vi "X_Limit_Length_Key_Down.vi"(1 "Max String Length":i32, 2 "Char":i16, 3 "Input String":string) -> (0 "Discard?":bool)   [LabVIEW 2012, in "String_XControl.xctl"]
doc: "This code takes in the last char pressed, the maximum string length, and the current string. The output is a boolean that indicates whether or not to discard the last key press."
uses:
  String_XControl.xctl
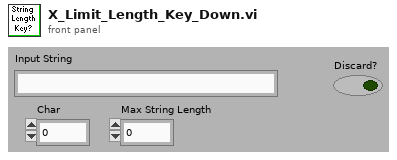
[diagram p1: front panel]
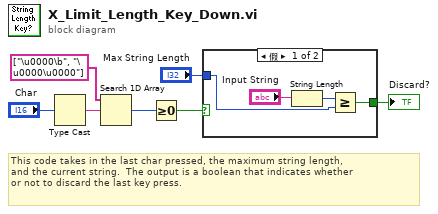
[diagram p0: block diagram]
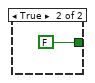
[diagram p2: hidden frame]
diagram:
  # "This code takes in the last char pressed, the maximum string length,\nand the current string.  The output is a boolean that indicates whether\nor not to discard the last key press."
  n1 = Type Cast(x="Char") -> (*(type *) &x=w6:string)  [unwired: 1 out]
  n2 = Search 1D Array(1D array=string[] ["\u0000\b", "\u0000\u0000"], element=w6) -> (index of element=w2:i32)  [unwired: 1 out]
  n3 = Greater Or Equal To 0?(x=w2) -> (x >= 0?=w4:bool)
  n4 = case shown="假" w4 {
    tunnel: [w9 FALSE] -> w3
    tunnel: "Max String Length" -> [w8 _]
    frame False {
      n5 = String Length(string="Input String") -> (length=w10:i32)
      n6 = Greater Or Equal?(x=w10, y=w8) -> (x >= y?=w9:bool)
    }
    frame True {
    }
  }
  "Discard?" <- w3
